vi "daq init.vi"(8 "error in":errorcluster, 10 "rate":dbl=25000.0 format="%0.2f", 11 "number of samples":i32=25000) -> (0 "error out":errorcluster, 3 "task out":refnum<k21>)   [LabVIEW 2013]
uses:
  <vilib>/DAQmx/configure/timing.llb/DAQmx Timing (Sample Clock).vi
  <vilib>/DAQmx/create/channels.llb/DAQmx Create Channel (AI-Voltage-Basic).vi
  <vilib>/DAQmx/create/channels.llb/DAQmx Create Channel (TEDS-AI-Voltage-Basic).vi
  <vilib>/DAQmx/create/channels.llb/DAQmx Create Channel (TEDS-AI-Current-Basic).vi
  <vilib>/DAQmx/create/channels.llb/DAQmx Create Channel (AI-Current-Basic).vi
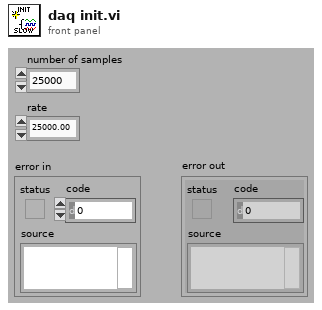
[diagram p1: front panel]
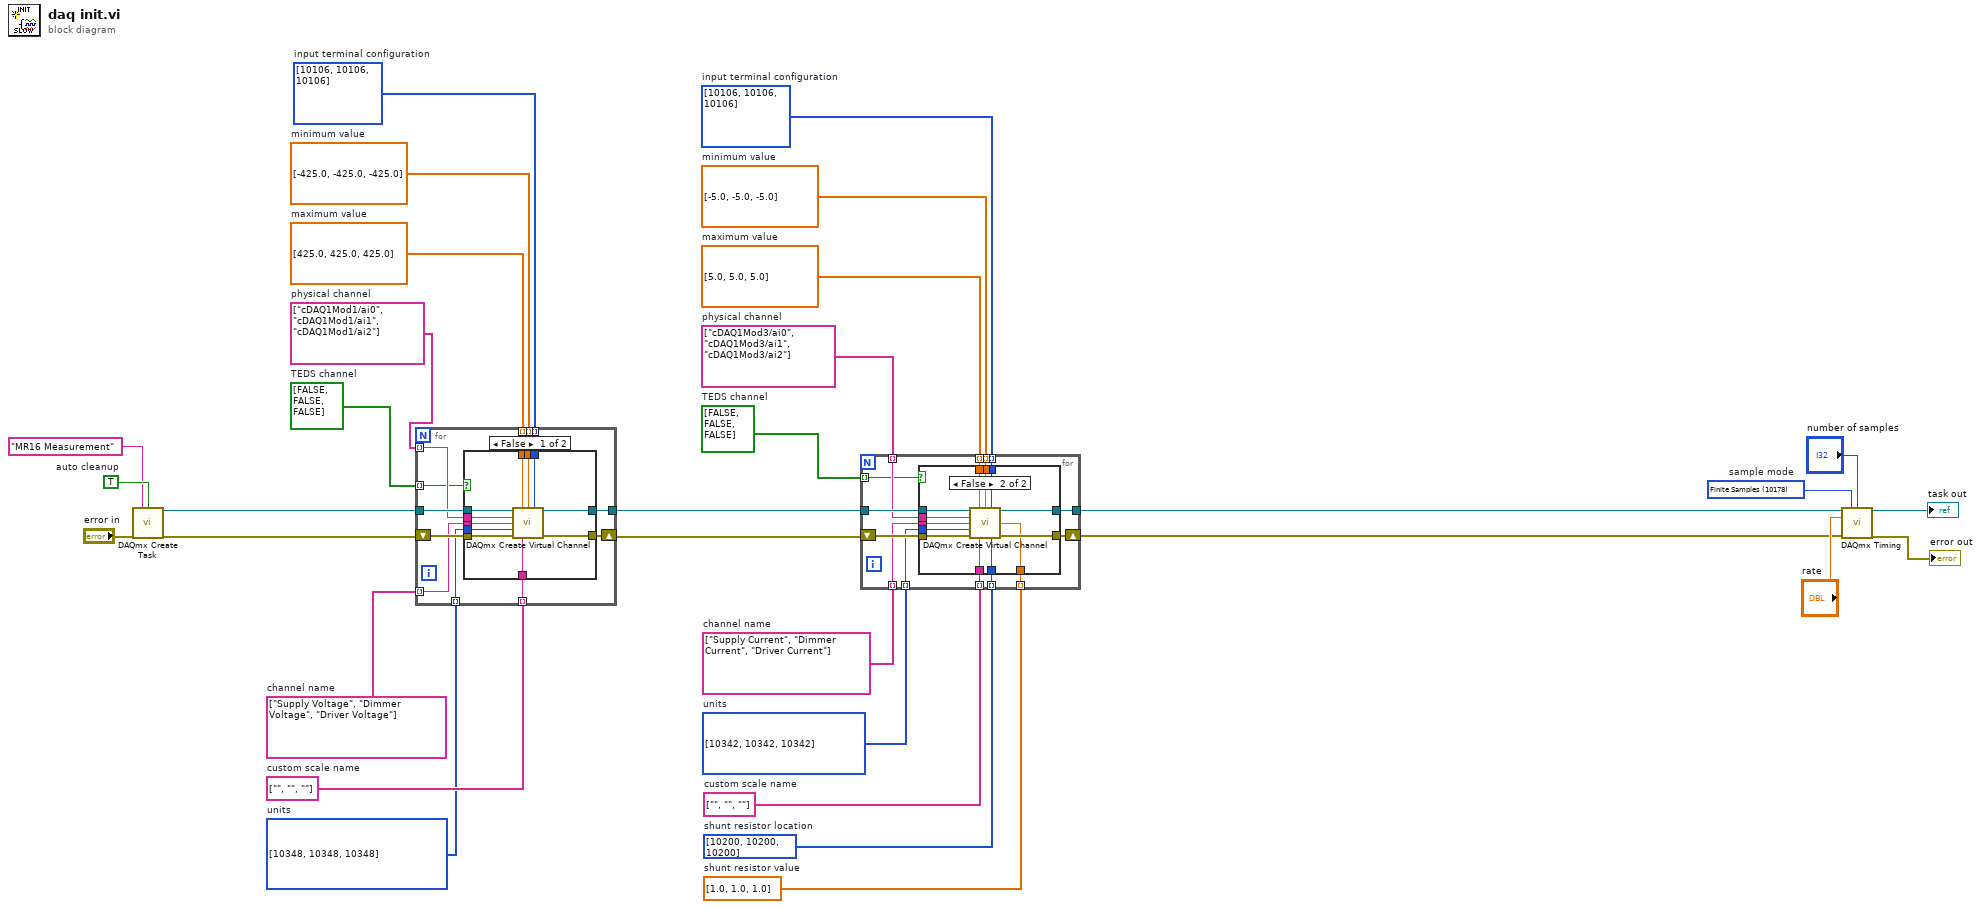
[diagram p0: block diagram]
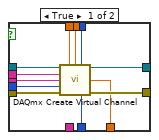
[diagram p2: hidden frame]
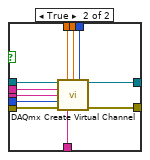
[diagram p3: hidden frame]
diagram:
  w3 = string[] ["", "", ""]  # custom scale name
  w5 = 10178 items=["Finite Samples"=10178, "Continuous Samples"=10123, "Hardware Timed Single Point"=12522]  # sample mode
  w10 = bool[] [FALSE, FALSE, FALSE]  # TEDS channel
  w12 = i32[] [10200, 10200, 10200] items=["Internal"=10200, "External"=10167]  # shunt resistor location
  w11 = dbl[] [1.0, 1.0, 1.0]  # shunt resistor value
  w15 = i32[] [10342, 10342, 10342] items=["Amps"=10342, "From TEDS"=12516, "From Custom Scale"=10065]  # units
  w14 = string[] ["Supply Current", "Dimmer Current", "Driver Current"]  # channel name
  w13 = string[] ["cDAQ1Mod3/ai0", "cDAQ1Mod3/ai1", "cDAQ1Mod3/ai2"]  # physical channel
  w16 = dbl[] [5.0, 5.0, 5.0]  # maximum value
  w17 = dbl[] [-5.0, -5.0, -5.0]  # minimum value
  w18 = i32[] [10106, 10106, 10106] items=["default"=-1, "RSE"=10083, "NRSE"=10078, "Differential"=10106, "Pseudodifferential"=12529]  # input terminal configuration
  w20 = bool[] [FALSE, FALSE, FALSE]  # TEDS channel
  w25 = string[] ["", "", ""]  # custom scale name
  w24 = i32[] [10348, 10348, 10348] items=["Volts"=10348, "From TEDS"=12516, "From Custom Scale"=10065]  # units
  w23 = string[] ["Supply Voltage", "Dimmer Voltage", "Driver Voltage"]  # channel name
  w22 = string[] ["cDAQ1Mod1/ai0", "cDAQ1Mod1/ai1", "cDAQ1Mod1/ai2"]  # physical channel
  w26 = dbl[] [425.0, 425.0, 425.0]  # maximum value
  w27 = dbl[] [-425.0, -425.0, -425.0]  # minimum value
  w28 = i32[] [10106, 10106, 10106] items=["default"=-1, "RSE"=10083, "NRSE"=10078, "Differential"=10106, "Pseudodifferential"=12529]  # input terminal configuration
  w30 = TRUE  # auto cleanup
  n1 = call <vilib>:"DAQmx Create Task.vi"("new task name"="MR16 Measurement", "auto cleanup"=w30, "error in"="error in") -> ("task out"=w29:refnum<k21>, "error out"=w31:errorcluster)  [unwired: 11 in]
  n2 = for {
    tunnel: w29 -> [w41]
    tunnel: w28 -> [w42] mode=indexing
    tunnel: w27 -> [w43] mode=indexing
    tunnel: w26 -> [w44] mode=indexing
    tunnel: w25 -> [w34] mode=indexing
    tunnel: w24 -> [w35] mode=indexing
    tunnel: w23 -> [w37] mode=indexing
    tunnel: w22 -> [w36] mode=indexing
    tunnel: [w39] -> w19
    shift-right: [w38] -> w21
    shift-left: w31 -> [w40]
    tunnel: w20 -> [w33] mode=indexing
    n3 = case shown="False" w33 {
      tunnel: w44 -> [w55 w60]
      tunnel: w43 -> [w54 w61]
      tunnel: w42 -> [w53 w62]
      tunnel: w41 -> [w52 w66]
      tunnel: w40 -> [w51 w65]
      tunnel: [w50 w63] -> w39
      tunnel: [w49 w64] -> w38
      tunnel: w37 -> [w48 w58]
      tunnel: w36 -> [w47 w59]
      tunnel: w35 -> [w46 w57]
      tunnel: w34 -> [w45 w56]
      frame False {
        n4 = call-poly <vilib>:"DAQmx Create Virtual Channel.vi"("task in"=w52, "maximum value"=w55, "minimum value"=w54, "input terminal configuration"=w53, "physical channels"=w47, "name to assign"=w48, "units"=w46, "error in"=w51, "custom scale name"=w45) -> ("task out"=w50:refnum<k21>, "error out"=w49:errorcluster)  [unwired: 5 in]
      }
      frame True {
        n5 = call-poly <vilib>:"DAQmx Create Virtual Channel.vi"("task in"=w66, "maximum value"=w60, "minimum value"=w61, "input terminal configuration"=w62, "physical channels"=w59, "name to assign"=w58, "units"=w57, "error in"=w65, "custom scale name"=w56) -> ("task out"=w63:refnum<k21>, "error out"=w64:errorcluster)  [unwired: 5 in]
      }
    }
  }
  n6 = for {
    tunnel: w19 -> [w77]
    tunnel: w18 -> [w80] mode=indexing
    tunnel: w17 -> [w79] mode=indexing
    tunnel: w16 -> [w78] mode=indexing
    tunnel: w15 -> [w71] mode=indexing
    tunnel: w14 -> [w73] mode=indexing
    tunnel: w13 -> [w72] mode=indexing
    tunnel: [w75] -> w2
    tunnel: w12 -> [w70] mode=indexing
    tunnel: w11 -> [w69] mode=indexing
    shift-right: [w74] -> w1
    shift-left: w21 -> [w76]
    tunnel: w10 -> [w68] mode=indexing
    tunnel: w3 -> [w67] mode=indexing
    n7 = case shown="False" w68 {
      tunnel: w80 -> [w92 w105]
      tunnel: w79 -> [w91 w104]
      tunnel: w78 -> [w90 w103]
      tunnel: w77 -> [w89 w102]
      tunnel: w76 -> [w88 w101]
      tunnel: [w87 w100] -> w75
      tunnel: [w86 w99] -> w74
      tunnel: w73 -> [w85 w98]
      tunnel: w72 -> [w84 w97]
      tunnel: w71 -> [w83 w96]
      tunnel: w70 -> [w82 w95]
      tunnel: w69 -> [w81 w94]
      tunnel: w67 -> [_ w93]
      frame True {
        n8 = call-poly <vilib>:"DAQmx Create Virtual Channel.vi"("task in"=w89, "maximum value"=w90, "minimum value"=w91, "input terminal configuration"=w92, "physical channels"=w84, "name to assign"=w85, "external shunt resistor value"=w81, "units"=w83, "error in"=w88, "shunt resistor location"=w82) -> ("task out"=w87:refnum<k21>, "error out"=w86:errorcluster)  [unwired: 4 in]
      }
      frame False {
        n9 = call-poly <vilib>:"DAQmx Create Virtual Channel.vi"("task in"=w102, "maximum value"=w103, "minimum value"=w104, "input terminal configuration"=w105, "physical channels"=w97, "name to assign"=w98, "external shunt resistor value"=w94, "units"=w96, "error in"=w101, "custom scale name"=w93, "shunt resistor location"=w95) -> ("task out"=w100:refnum<k21>, "error out"=w99:errorcluster)  [unwired: 3 in]
      }
    }
  }
  n10 = call-poly <vilib>:"DAQmx Timing.vi"("task/channels in"=w2, "sample mode"=w5, "samples per channel"="number of samples", "rate"="rate", "error in"=w1) -> ("task out"=→"task out":refnum<k21>, "error out"=→"error out":errorcluster)  [unwired: 9 in]
